vi "Teleop.vi"(10 "Match Info":T3={"Autonomous Elapsed Seconds"=0.0, "TeleOp Elapsed Seconds"=0.0, "Disabled Elapsed Seconds"=0.0, "Visited Autonomous"=FALSE, "Visited TeleOp"=FALSE, "Visited Disabled"=FALSE, "Autonomous Settings"={"Autonomous Style"=enum."Independent", "VI Refnum"=refnum}}, 11 "Call Context":T4) -> ()   [LabVIEW 2020]
doc: "This VI is called for each TeleOp packet received from the DS where the robot is not disabled. It is often used to read from the joysticks and update I/O or to update setpoints for timed control loops. It should complete and return within 20 milliseconds or it may miss DS packets."
uses:
  <vilib>/Rock Robotics/WPI/DriverStation/WPI_DriverStationDerivedRobotMode.ctl
  <vilib>/Rock Robotics/WPI/DriverStation/WPI_DriverStationMatch Info.ctl
  <vilib>/Rock Robotics/WPI/Solenoid/WPI_SolenoidValue.ctl
  <vilib>/Rock Robotics/WPI/ThirdParty/Phoenix-LabVIEW/Motor Controller/Controls/CTRE_Phoenix_MotorControl_ControlMode.ctl
  <vilib>/Rock Robotics/WPI/Utilities/WPI_GetSetVariantRefNum.vi
  <vilib>/Rock Robotics/WPI/ThirdParty/Phoenix-LabVIEW/Pigeon IMU/CTRE_PigeonIMU_GetYPR.vi
  <vilib>/Rock Robotics/Network Tables/NT Read Boolean.vi
  <vilib>/Rock Robotics/Network Tables/NT Read Number.vi
  <vilib>/Rock Robotics/Network Tables/NT Read String.vi
  <vilib>/Rock Robotics/Network Tables/NT Write Boolean.vi
  <vilib>/Rock Robotics/WPI/ThirdParty/Phoenix-LabVIEW/CANCoder/Get/CTRE_Phoenix_CANcoder_GetSensorData.vi
  <vilib>/Rock Robotics/Network Tables/NT Write String.vi
  <vilib>/Rock Robotics/WPI/Solenoid/WPI_SolenoidSetEnum.vi
  <vilib>/Rock Robotics/WPI/ThirdParty/Phoenix-LabVIEW/Motor Controller/Get/CTRE_Phoenix_MotorController_IntegratedSensorData_TalonFX.vi
  <vilib>/addons/control/pid/pid.llb/PID (DBL).vi
  <vilib>/addons/control/pid/NI_PID_pid.lvlib
panel:
  out "reject pressed":bool
  out "intake count":i32
  in  "Subtract rpm":dbl=2700.0
  out "% voltage":dbl
  out "voltage (V)":dbl
  out "Motor Volts":dbl
  out "rpm":dbl
  in  "intake start":T1=enum."Forward"
  out "limelight tx":dbl
  out "limelight ty":dbl
  in  "Elevate no want":dbl
  in  "Reject no want":dbl=-1.0
  in  "Intake no want":dbl=0.75 format="%#_13g"
  in  "Elevate wanted":dbl=-0.35
  in  "Reject wanted":dbl=1.0
  in  "Intake wanted":dbl=0.75
  out "Pigeon Value":dbl
  out "frontrightmotor":dbl
  out "frontleftdrive":dbl
  in  "PID gains 4":T2={"proportional gain (Kc)"=-0.005, "integral time (Ti, min)"=0.0, "derivative time (Td, min)"=2e-05} {"derivative time (Td, min)" format="%.6f"; "integral time (Ti, min)" format="%.6f"; "proportional gain (Kc)" format="%.6f"}
  in  "PID gains 3":T2={"proportional gain (Kc)"=0.005, "integral time (Ti, min)"=0.0, "derivative time (Td, min)"=2e-05} {"derivative time (Td, min)" format="%.6f"; "integral time (Ti, min)" format="%.6f"; "proportional gain (Kc)" format="%.6f"}
  in  "PID gains 2":T2={"proportional gain (Kc)"=-0.005, "integral time (Ti, min)"=0.0, "derivative time (Td, min)"=2e-05} {"derivative time (Td, min)" format="%.6f"; "integral time (Ti, min)" format="%.6f"; "proportional gain (Kc)" format="%.6f"}
  in  "PID gains":T2={"proportional gain (Kc)"=0.005, "integral time (Ti, min)"=0.0, "derivative time (Td, min)"=2e-05} {"derivative time (Td, min)" format="%.6f"; "integral time (Ti, min)" format="%.6f"; "proportional gain (Kc)" format="%.6f"}
  out "Motor out 4":dbl
  out "Desired Position 4":dbl
  out "Motor out 1":dbl
  out "Desired Position 1":dbl
  out "Motor Out 2":dbl
  out "Desired Position 2":dbl
  out "Motor out 3":dbl
  out "Desired Position 3":dbl
  out "Sensor Position 4":dbl
  out "Sensor Position 3":dbl
  out "Sensor Position 2":dbl
  out "Sensor Position 1":dbl
  out "Rotation steering angle 4":dbl
  out "WheelDirection4":dbl(knob) scale=180.0..-180.0
  out "Throttle 4":dbl(slide) scale=-1.0..1.0
  out "Y4":dbl
  out "X4":dbl
  out "Rotation steering angle 3":dbl
  out "WheelDirection3":dbl(knob) scale=180.0..-180.0
  out "Throttle 3":dbl(slide) scale=-1.0..1.0
  out "Y3":dbl
  out "X3":dbl
  out "Rotation steering angle 2":dbl
  out "WheelDirection2":dbl(knob) scale=180.0..-180.0
  out "Throttle 2":dbl(slide) scale=-1.0..1.0
  out "Y2":dbl
  out "X2":dbl
  out "Rotation steering angle 1":dbl
  out "WheelDirection1":dbl(knob) scale=180.0..-180.0
  out "Throttle 1":dbl(slide) scale=-1.0..1.0
  out "Y1":dbl
  out "X1":dbl
  out "Z - Axis":dbl
  out "Y - Axis":dbl
  out "X - Axis":dbl
  in  "Auto-Accept":bool
  in  "8togglePressed?":bool
  in  "Red/Blue":u32(colorbox)
  out "B":u8
  out "G":u8
  out "R":u8
  out "Color":u32(colorbox)
  out "Sample Slider 0":dbl(slide) scale=0.0..5.0
  out "Sample Boolean 1":bool
  out "Sample Boolean 0":bool
  # "-1"
  # "0"
  # ".75"
  # ".75"
  # "-.6"
  # "-.35"
  # ".1"
  # "1"
  # "-.1"
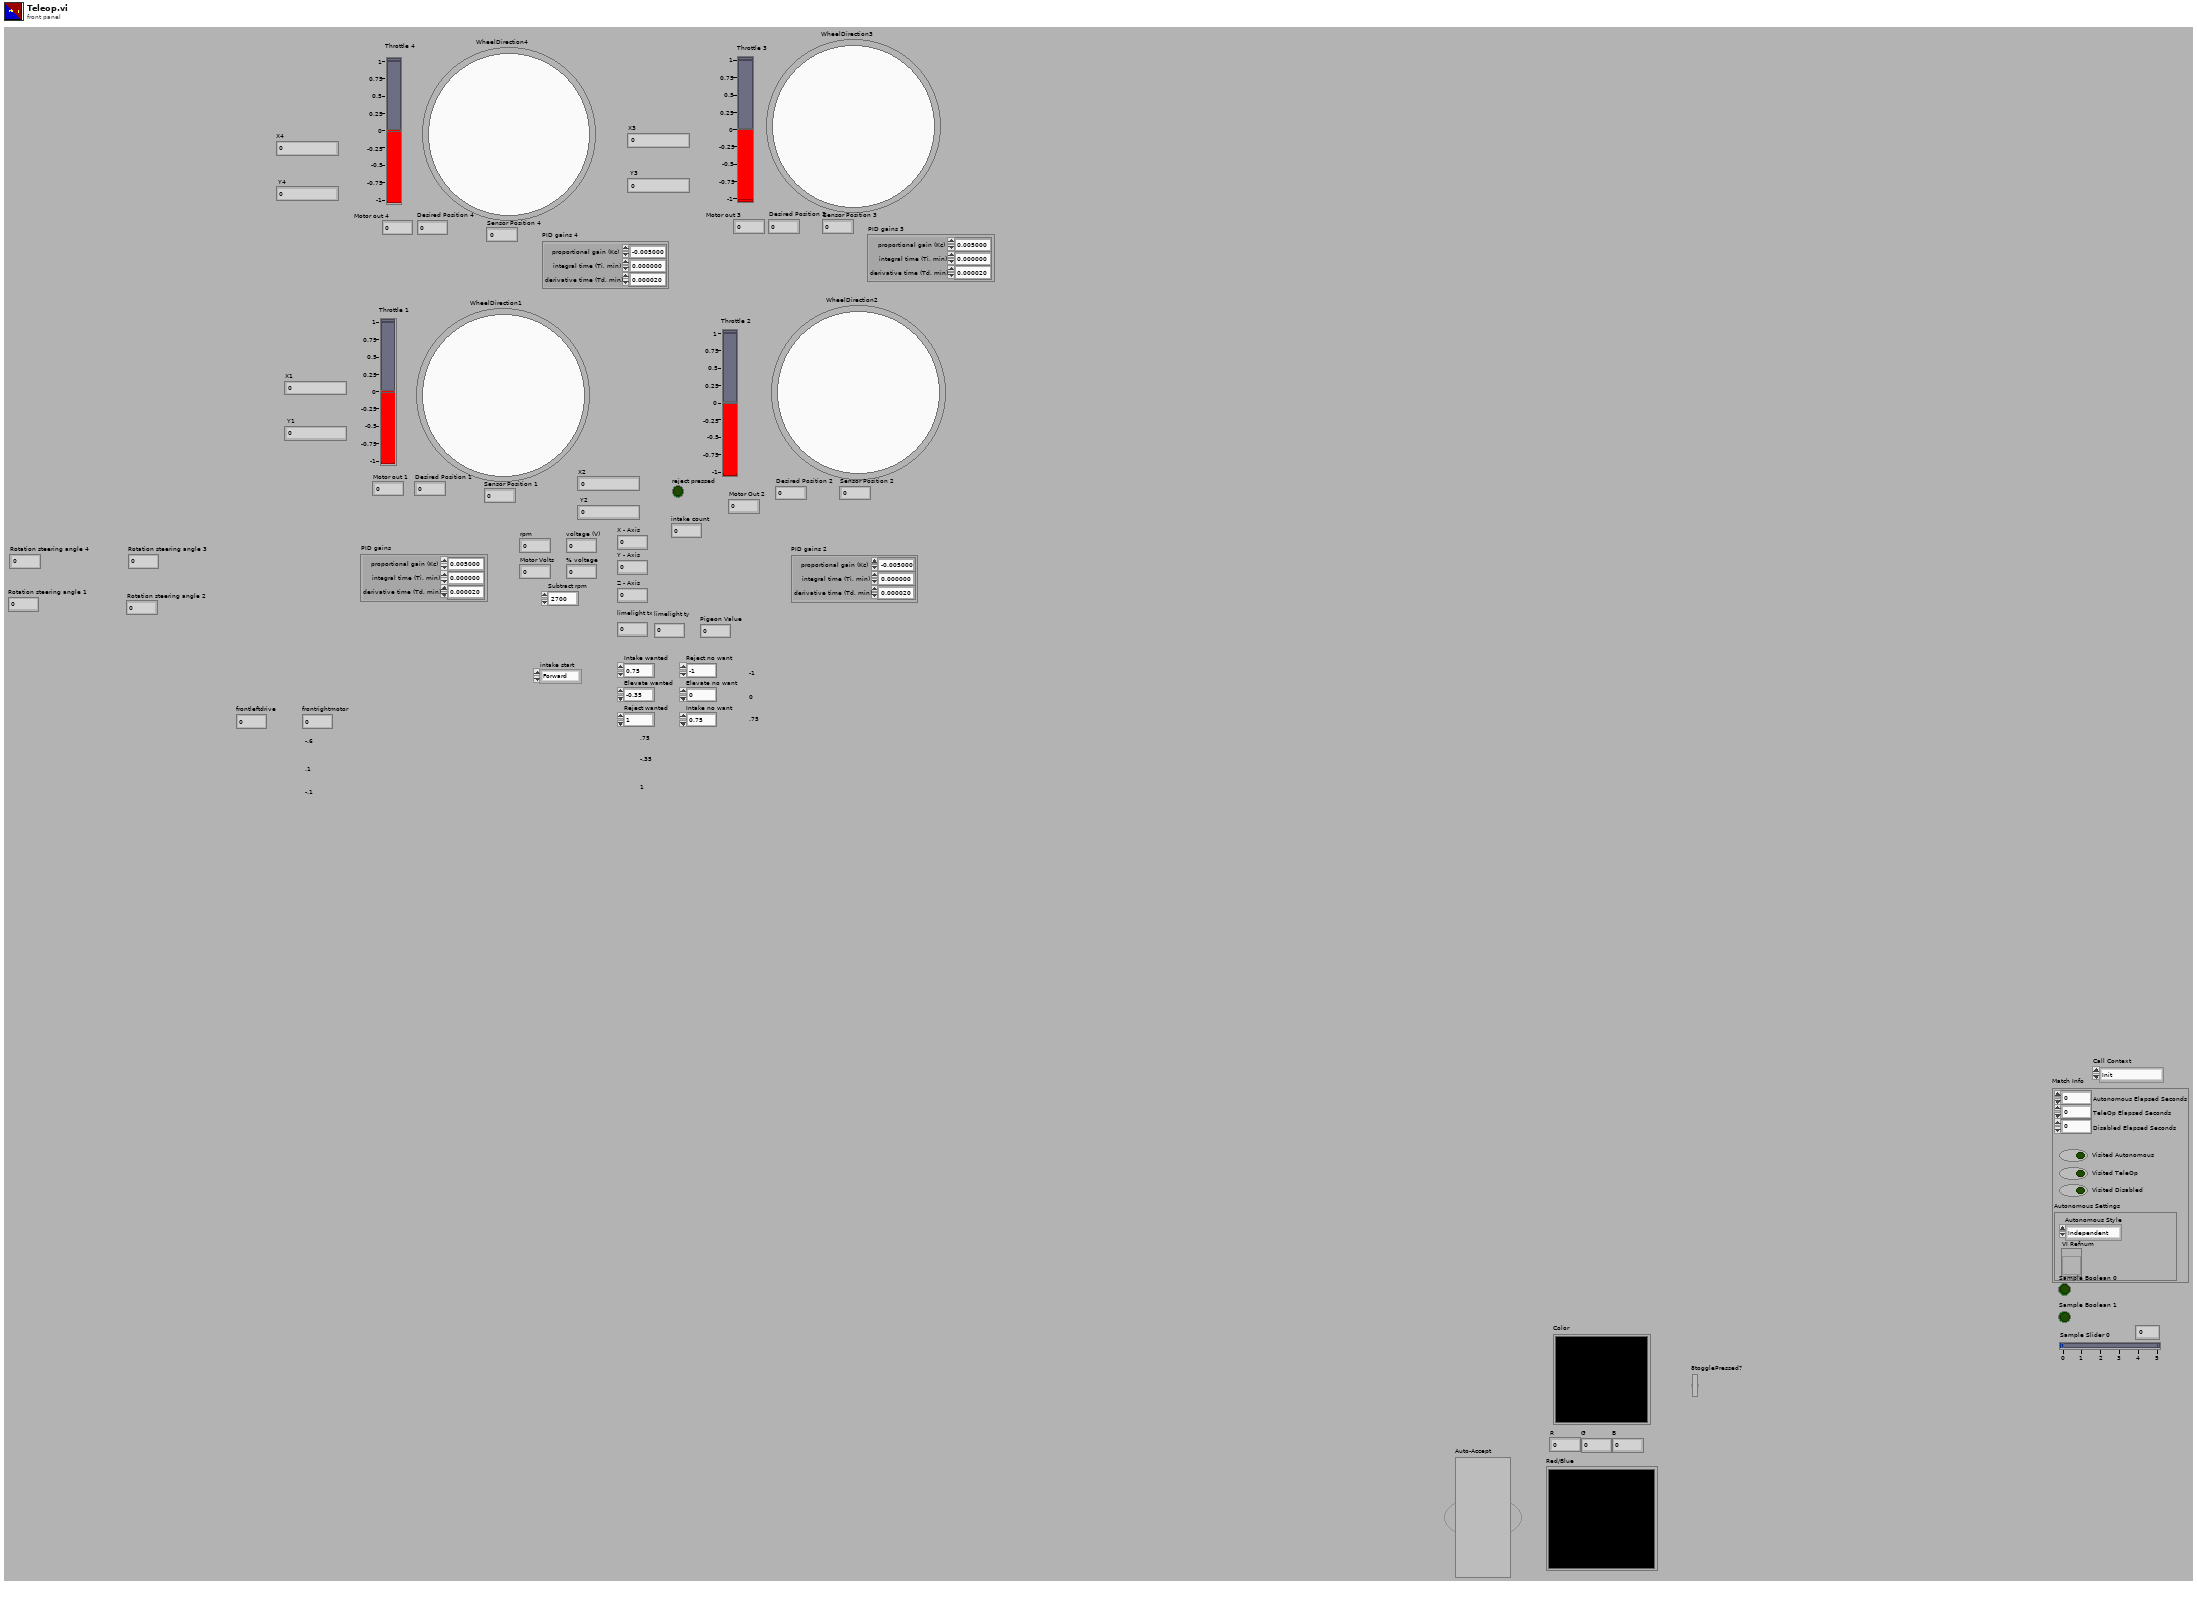
[diagram p1: front panel]
types:
  T1 = typedef "WPI_SolenoidValue.ctl" = enum16{"Off", "On", "Forward", "Reverse"}
  T2 = cluster{"proportional gain (Kc)":dbl, "integral time (Ti, min)":dbl, "derivative time (Td, min)":dbl}
  T3 = typedef "WPI_DriverStationMatch Info.ctl" = cluster{"Autonomous Elapsed Seconds":dbl, "TeleOp Elapsed Seconds":dbl, "Disabled Elapsed Seconds":dbl, "Visited Autonomous":bool, "Visited TeleOp":bool, "Visited Disabled":bool, "Autonomous Settings":cluster{"Autonomous Style":enum16{"Iterative", "Independent"}, "VI Refnum":refnum<vi>}}
  T4 = typedef "WPI_DriverStationDerivedRobotMode.ctl" = enum16{"Init", "Execute", "Stop"}
  T5 = typedef "CTRE_Phoenix_MotorControl_ControlMode.ctl" = u16
  T6 = typedef "WPI_MotorControlDeviceRef.ctl" = cluster{"DeviceStatus":errorcluster, "Type":T7, "PWM":cluster{"PWM Channel":T8, "DeadBand":T9}, "CAN":cluster{"Device Number":u8, "SetOutput VI Ref":variant, "GetOutput VI Ref":variant, "Enable VI Ref":variant, "Disable VI Ref":variant, "Data":variant}, "Invert":bool, "DIO PWM":cluster{"PWM \"Enable\" Channel":T8, "DIOChannel":T10, "PWM Rate":dbl}}
  T7 = typedef "WPI_MotorControlType.ctl" = enum16{"PWM", "CAN", "DIO PWM"}
  T8 = typedef "FPGA_DIOPWMChannel.ctl" = enum8{"PWM 0", "PWM 1", "PWM 2", "PWM 3", "PWM 4", "PWM 5", "PWM 6", "PWM 7", "PWM 8", "PWM 9", "PWM MXP 0", "PWM MXP 1", "PWM MXP 2", "PWM MXP 3", "PWM MXP 4", "PWM MXP 5", "PWM MXP 6", "PWM MXP 7", "PWM MXP 8", "PWM MXP 9", "Invalid"}
  T9 = typedef "WPI_PWMDeadband.ctl" = cluster{"Name":string, "maxPositivePwm":i32, "minPositivePwm":i32, "centerPwm":i32, "maxNegativePwm":i32, "minNegativePwm":i32, "angularRange":u16}
  T10 = typedef "FPGA_DIOChannel.ctl" = enum8{"DIO 0", "DIO 1", "DIO 2", "DIO 3", "DIO 4", "DIO 5", "DIO 6", "DIO 7", "DIO 8", "DIO 9", "DIO MXP 0", "DIO MXP 1", "DIO MXP 2", "DIO MXP 3", "DIO MXP 4", "DIO MXP 5", "DIO MXP 6", "DIO MXP 7", "DIO MXP 8", "DIO MXP 9", "DIO MXP 10", "DIO MXP 11", "DIO MXP 12", "DIO MXP 13", "DIO MXP 14", "DIO MXP 15", "SPI Port CS1", "SPI Port CS2", "SPI Port CS3", "SPI Port MISO", "SPI Port MOSI", "Invalid"}
  T11 = typedef "WPI_SolenoidDevRef.ctl" = cluster{"DevStatus":errorcluster, "Pneumatics Control Module":u8, "Forward Solenoid Channel":T12, "Reverse Solenoid Channel":T12}
  T12 = typedef "WPI_SolenoidChannel.ctl" = enum8{"Solenoid 0", "Solenoid 1", "Solenoid 2", "Solenoid 3", "Solenoid 4", "Solenoid 5", "Solenoid 6", "Solenoid 7", "Solenoid 8", "Solenoid 9", "Solenoid 10", "Solenoid 11", "Solenoid 12", "Solenoid 13", "Solenoid 14", "Solenoid 15", "Invalid"}
  T13 = typedef "WPI_CompressorDevRef.ctl" = cluster{"DevStatus":errorcluster, "Pneumatics Control Module":u8}
  T14 = typedef "WPI_SwitchDevRef.ctl" = cluster{"DevStatus":errorcluster, "DIO Channel":T10, "CntIndex":T15, "Normally Closed":bool}
  T15 = typedef "FPGA_CounterCtrSystemIndex.ctl" = enum8{"Ctr 0", "Ctr 1", "Ctr 2", "Ctr 3", "Ctr 4", "Ctr 5", "Ctr 6", "Ctr 7", "Invalid"}
  T16 = typedef "Color Sensor V3 DevRef.ctl" = cluster{"I2CDevRef":T17}
  T17 = typedef "WPI_I2CDevRef.ctl" = cluster{"DevStatus":errorcluster, "Device Address":u8, "Handle":i32, "I2C Bus":T18}
  T18 = typedef "i2c_bus.ctl" = enum16{"I2C On-Board", "I2C MXP", "Invalid"}
  T19 = typedef "WPI_JoystickDevRef.ctl" = cluster{"Device":T20}
  T20 = typedef "WPI_JoystickDeviceEnum.ctl" = enum16{"USB 0", "USB 1", "USB 2", "USB 3", "USB 4", "USB 5"}
  T21 = typedef "CTRE_PigeonIMU_DeviceRef.ctl" = cluster{"DeviceStatus":errorcluster, "Device Number":u8, "Type":T22, "Device ID":u32, "Handle":u64, "UsageFrame":u32, "Library Path":path}
  T22 = typedef "CTRE_PigeonIMU_ConnectionType.ctl" = u32
  T23 = typedef "CTRE_Phoenix_CANcoder_DeviceRef.ctl" = cluster{"DeviceStatus":errorcluster, "Device Number":u8, "Handle":u64, "UsageFrame":u32, "Library Path":path}
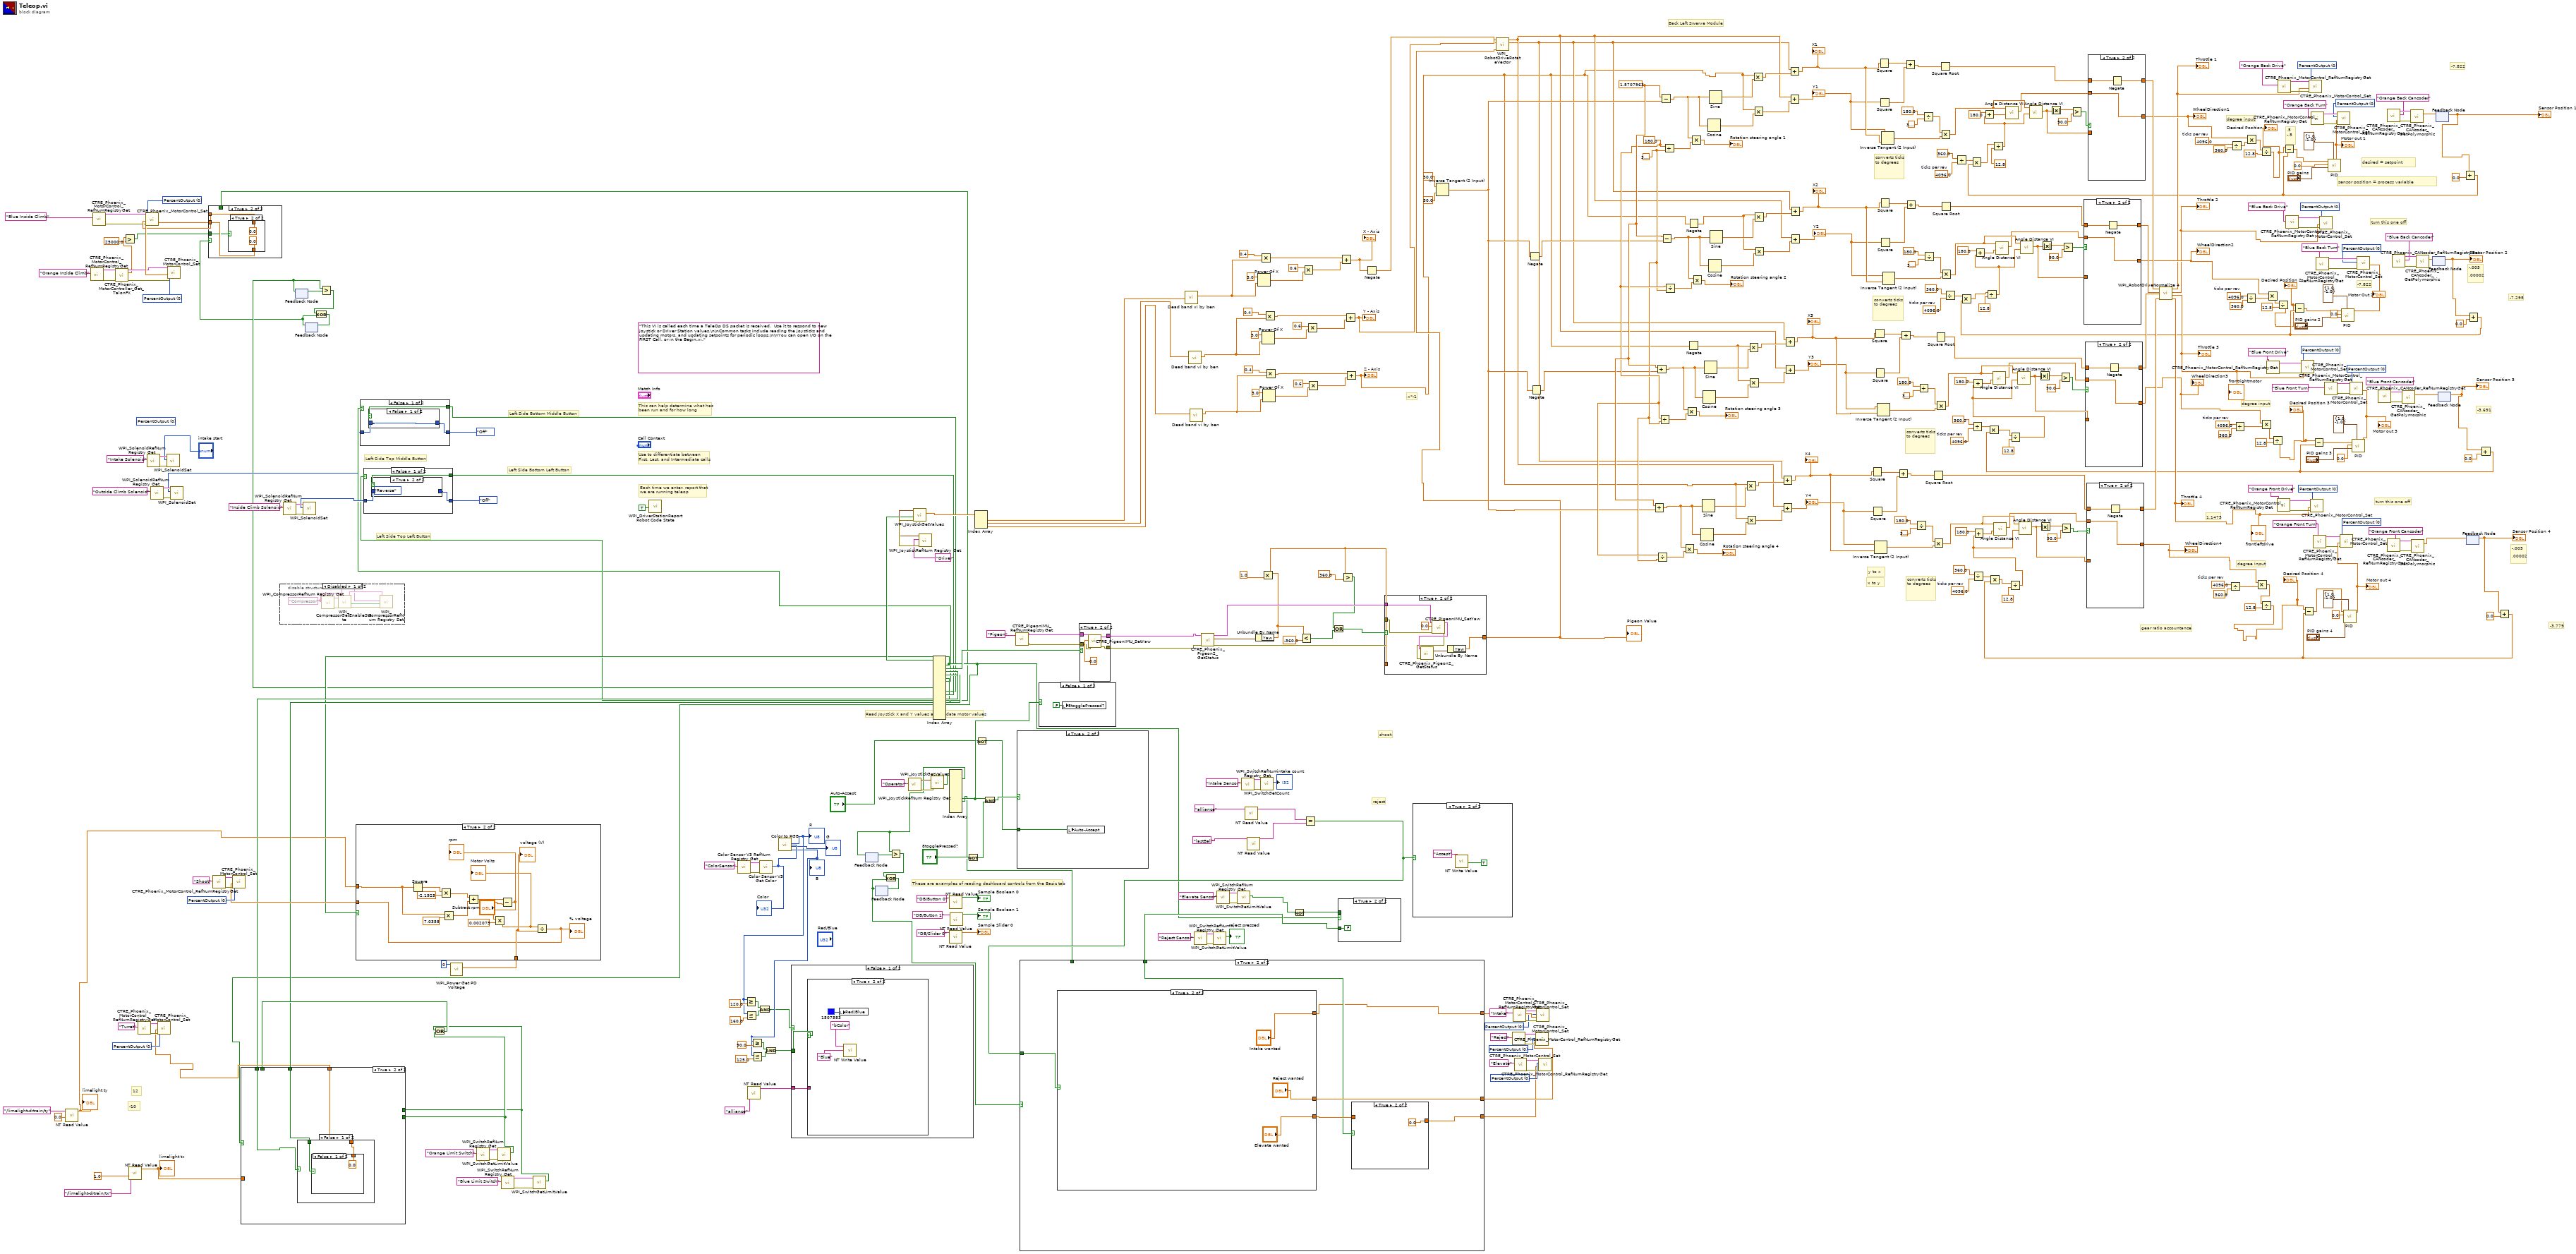
[diagram p0: block diagram]
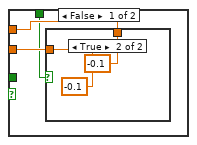
[diagram p2: hidden frame]
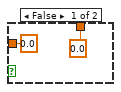
[diagram p3: hidden frame]
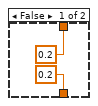
[diagram p4: hidden frame]
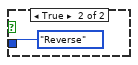
[diagram p6: hidden frame]
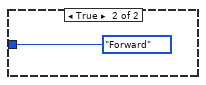
[diagram p7: hidden frame]
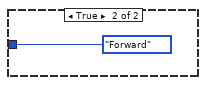
[diagram p9: hidden frame]
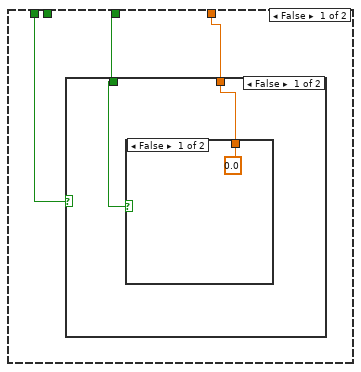
[diagram p10: hidden frame]
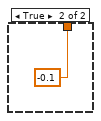
[diagram p11: hidden frame]
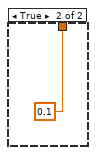
[diagram p12: hidden frame]
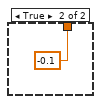
[diagram p13: hidden frame]
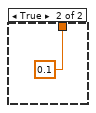
[diagram p14: hidden frame]
diagram:
  w18 = T5 0 items=["PercentOutput"=0, "Position"=1, "Velocity"=2, "Current"=3, "Follower"=5, "MotionProfile"=6, "MotionMagic"=7, "MotionProfileArc"=10, "Disabled"=15] ("Control Mode")
  w19 = T5 0 items=["PercentOutput"=0, "Position"=1, "Velocity"=2, "Current"=3, "Follower"=5, "MotionProfile"=6, "MotionMagic"=7, "MotionProfileArc"=10, "Disabled"=15] ("Control Mode")
  (unwired) T5 0 items=["PercentOutput"=0, "Position"=1, "Velocity"=2, "Current"=3, "Follower"=5, "MotionProfile"=6, "MotionMagic"=7, "MotionProfileArc"=10, "Disabled"=15] ("Control Mode")
  w88 = T5 0 items=["PercentOutput"=0, "Position"=1, "Velocity"=2, "Current"=3, "Follower"=5, "MotionProfile"=6, "MotionMagic"=7, "MotionProfileArc"=10, "Disabled"=15] ("Control Mode")
  w189 = T5 0 items=["PercentOutput"=0, "Position"=1, "Velocity"=2, "Current"=3, "Follower"=5, "MotionProfile"=6, "MotionMagic"=7, "MotionProfileArc"=10, "Disabled"=15] ("Control Mode")
  w201 = T5 0 items=["PercentOutput"=0, "Position"=1, "Velocity"=2, "Current"=3, "Follower"=5, "MotionProfile"=6, "MotionMagic"=7, "MotionProfileArc"=10, "Disabled"=15] ("Control Mode")
  w202 = T5 0 items=["PercentOutput"=0, "Position"=1, "Velocity"=2, "Current"=3, "Follower"=5, "MotionProfile"=6, "MotionMagic"=7, "MotionProfileArc"=10, "Disabled"=15] ("Control Mode")
  w203 = T5 0 items=["PercentOutput"=0, "Position"=1, "Velocity"=2, "Current"=3, "Follower"=5, "MotionProfile"=6, "MotionMagic"=7, "MotionProfileArc"=10, "Disabled"=15] ("Control Mode")
  w204 = T5 0 items=["PercentOutput"=0, "Position"=1, "Velocity"=2, "Current"=3, "Follower"=5, "MotionProfile"=6, "MotionMagic"=7, "MotionProfileArc"=10, "Disabled"=15] ("Control Mode")
  w205 = T5 0 items=["PercentOutput"=0, "Position"=1, "Velocity"=2, "Current"=3, "Follower"=5, "MotionProfile"=6, "MotionMagic"=7, "MotionProfileArc"=10, "Disabled"=15] ("Control Mode")
  w206 = T5 0 items=["PercentOutput"=0, "Position"=1, "Velocity"=2, "Current"=3, "Follower"=5, "MotionProfile"=6, "MotionMagic"=7, "MotionProfileArc"=10, "Disabled"=15] ("Control Mode")
  w207 = T5 0 items=["PercentOutput"=0, "Position"=1, "Velocity"=2, "Current"=3, "Follower"=5, "MotionProfile"=6, "MotionMagic"=7, "MotionProfileArc"=10, "Disabled"=15] ("Control Mode")
  w219 = 4096.0  # ticks per rev
  w231 = 4096.0  # ticks per rev
  w245 = 4096.0  # ticks per rev
  w256 = 4096.0  # ticks per rev
  w152 = 1.5707963 ("y")
  w265 = 4096.0  # ticks per rev
  w269 = 4096.0  # ticks per rev
  w273 = 4096.0  # ticks per rev
  w192 = 4096.0  # ticks per rev
  w150 = 3.141592653589793
  w151 = 180.0 ("x")
  w371 = T5 0 items=["PercentOutput"=0, "Position"=1, "Velocity"=2, "Current"=3, "Follower"=5, "MotionProfile"=6, "MotionMagic"=7, "MotionProfileArc"=10, "Disabled"=15] ("Control Mode")
  w387 = T5 0 items=["PercentOutput"=0, "Position"=1, "Velocity"=2, "Current"=3, "Follower"=5, "MotionProfile"=6, "MotionMagic"=7, "MotionProfileArc"=10, "Disabled"=15] ("Control Mode")
  w388 = T5 0 items=["PercentOutput"=0, "Position"=1, "Velocity"=2, "Current"=3, "Follower"=5, "MotionProfile"=6, "MotionMagic"=7, "MotionProfileArc"=10, "Disabled"=15] ("Control Mode")
  w392 = T5 0 items=["PercentOutput"=0, "Position"=1, "Velocity"=2, "Current"=3, "Follower"=5, "MotionProfile"=6, "MotionMagic"=7, "MotionProfileArc"=10, "Disabled"=15] ("Control Mode")
  (unwired) "This VI is called each time a TeleOp DS packet is received.  Use it to respond to new joystick or Driver Station values.\n\nCommon tasks include reading the joysticks and updating motors, and updating setpoints for periodic loops.\n\nYou can open I/O on the FIRST Call, or in the Begin.vi."
  # "Left Side Bottom Middle Button"
  # "Left Side Top Middle Button"
  # "Left Side Bottom Left Button"
  # "Left Side Top Left Button"
  # "shoot"
  # "reject"
  # "x*-1"
  # "12"
  # "-10"
  # ".5\n-.5"
  # "y to x"
  # "x to y"
  # "sensor position = process variable"
  # "desired = setpoint"
  # "-.005\n\n.00002"
  # "-.005\n\n.00002"
  # "-7.822"
  # "-7.295"
  # "-3.691"
  # "-3.779"
  # "1.1475"
  # "turn this one off"
  # "turn this one off"
  # "gear ratio accountance"
  # "converts ticks to degrees"
  # "converts ticks to degrees"
  # "converts ticks to degrees"
  # "converts ticks to degrees"
  # "degree input"
  # "degree input"
  # "degree input"
  # "Back Left Swerve Module"
  # "These are examples of reading dashboard controls from the Basic tab"
  # "Read Joystick X and Y values and update motor values"
  # "-7.822"
  # "Each time we enter, report that\nwe are running teleop"
  # "Use to differentiate between\nFirst, Last, and Intermediate calls"
  # "This can help determine what has\nbeen run and for how long"
  n1 = call-poly <vilib>:"NT Read Value.vi"("Default Value"=0.0, "Name"="/limelight-drtrain/ty") -> ("Numeric"=w38:dbl)  [unwired: 8 in, 1 out]
  "limelight ty" <- w38
  n2 = call <vilib>:"CTRE_Phoenix_MotorControl_RefNumRegistryGet.vi"("refnum name"="Orange Inside Climb") -> ("error out"=w15:errorcluster, "PhoenixMotorControlDevRef"=w14:T6)  [unwired: 9 in]
  n3 = call <vilib>:"CTRE_Phoenix_MotorControl_RefNumRegistryGet.vi"("refnum name"="Blue Inside Climb") -> ("error out"=w10:errorcluster, "PhoenixMotorControlDevRef"=w11:T6)  [unwired: 9 in]
  n4 = call-poly <vilib>:"CTRE_Phoenix_MotorController_Get_TalonFX.vi"("PhoenixMotorControlDevRef"=w14, "error in"=w15) -> ("PhoenixMotorControlDevRef"=w13:T6, "Position"=w3:dbl, "error out"=w12:errorcluster)  [unwired: 9 in, 2 out]
  n5 = Greater?(x=w3, y=25000.0) -> (0:w1:bool)
  n6 = call-poly <vilib>:"NT Read Value.vi"("Default Value"=1.0, "Name"="/limelight-drtrain/tx") -> ("Numeric"=w73:dbl)  [unwired: 8 in, 1 out]
  "limelight tx" <- w73
  n7 = call <vilib>:"CTRE_Phoenix_MotorControl_RefNumRegistryGet.vi"("refnum name"="Turret") -> ("error out"=w91:errorcluster, "PhoenixMotorControlDevRef"=w90:T6)  [unwired: 9 in]
  n8 = call <vilib>:"WPI_SolenoidRefNum Registry Get.vi"("refnum name"="Intake Solenoid") -> ("error out"=w77:errorcluster, "SolenoidDevRef"=w76:T11)  [unwired: 9 in]
  n9 = call <vilib>:"WPI_SolenoidRefNum Registry Get.vi"("refnum name"="Outside Climb Solenoid") -> ("error out"=w83:errorcluster, "SolenoidDevRef"=w82:T11)  [unwired: 9 in]
  n10 = call-poly <vilib>:"WPI_SolenoidSet.vi"("error in (no error)"=w77, "Value"="intake start", "SolenoidDevRef"=w76) -> ()  [unwired: 7 in, 2 out]
  n11 = call <vilib>:"CTRE_Phoenix_MotorControl_RefNumRegistryGet.vi"("refnum name"="Shoot") -> ("error out"=w374:errorcluster, "PhoenixMotorControlDevRef"=w373:T6)  [unwired: 9 in]
  n12 = disable-structure shown="Disabled" {
    frame Disabled {
      w449 = "Compressor" ("refnum name")
      n13 = call <vilib>:"WPI_CompressorRefNum Registry Get.vi"("refnum name"=w449) -> ("error out"=w454:errorcluster, "CompressorDevRef"=w453:T13)  [unwired: 9 in]
      n14 = call <vilib>:"WPI_CompressorGetEnableState.vi"("error in (no error)"=w454, "CompressorDevRef"=w453) -> ("error out"=w452:errorcluster, "Compressor Running"=w451:bool, "CompressorDevRef"=w450:T13)  [unwired: 3 in, 4 out]
      n15 = call <vilib>:"WPI_CompressorRefNum Registry Set.vi"("error in (no error)"=w452, "Test Mode Only"=w451, "refnum name"=w449, "CompressorDevRef"=w450) -> ()  [unwired: 6 in, 2 out]
    }
    frame Enabled {
    }
  }
  n16 = call <vilib>:"WPI_SolenoidRefNum Registry Get.vi"("refnum name"="Inside Climb Solenoid") -> ("error out"=w80:errorcluster, "SolenoidDevRef"=w79:T11)  [unwired: 9 in]
  n17 = feedback #1() -> (w9:bool)  [unwired: 1 in]
  n18 = feedback #2() -> (w5:bool)  [unwired: 1 in]
  n19 = call <vilib>:"WPI_Power Get PD Voltage.vi"("Power Distribution Panel (def)"=u8 0) -> ("voltage (V)"=w56:dbl)  [unwired: 13 in, 1 out]
  n20 = call <vilib>:"WPI_SwitchRefNum Registry Get.vi"("refnum name"="Orange Limit Switch") -> ("error out"=w72:errorcluster, "SwitchDevRef"=w71:T14)  [unwired: 9 in]
  n21 = call <vilib>:"WPI_SwitchGetLimitValue.vi"("error in (no error)"=w72, "SwitchDevRef"=w71) -> ("Switch Pressed"=w66:bool)  [unwired: 7 in, 2 out]
  n22 = call <vilib>:"WPI_SwitchRefNum Registry Get.vi"("refnum name"="Blue Limit Switch") -> ("error out"=w69:errorcluster, "SwitchDevRef"=w68:T14)  [unwired: 9 in]
  n23 = call <vilib>:"WPI_SwitchGetLimitValue.vi"("error in (no error)"=w69, "SwitchDevRef"=w68) -> ("Switch Pressed"=w65:bool)  [unwired: 7 in, 2 out]
  n24 = Or(x=w65, y=w66) -> (x .or. y?=w74:bool)
  n25 = call <vilib>:"WPI_DriverStationReport Robot Code State.vi"("TeleOp"=TRUE ("Autonomous")) -> ()  [unwired: 10 in, 1 out]
  n26 = call <vilib>:"Color Sensor V3 RefNum Registry Get.vi"("refnum name"="ColorSensor") -> ("error out"=w426:errorcluster, "ColorSensorDevRef"=w427:T16)  [unwired: 9 in]
  n27 = call-poly <vilib>:"NT Read Value.vi"("Name"="alliance") -> ("String"=w111:string)  [unwired: 9 in, 1 out]
  n28 = call <vilib>:"Color Sensor V3 Get Color.vi"("error in (no error)"=w426, "ColorSensorDevRef"=w427) -> ("Color"=w425:u32)  [unwired: 6 in, 3 out]
  "Color" <- w425
  n29 = call <vilib>:"Color to RGB.vi"("Color"=w425) -> ("R"=w419:u8, "G"=→"G":u8, "B"=w414:u8)  [unwired: 1 out]
  "R" <- w419
  "B" <- w414
  n30 = Greater Or Equal?(x=w419, y=120.0) -> (x >= y?=w422:bool)
  n31 = Less Or Equal?(x=w419, y=160.0) -> (x <= y?=w423:bool)
  n32 = Greater Or Equal?(x=w414, y=90.0) -> (x >= y?=w417:bool)
  n33 = Less Or Equal?(x=w414, y=125.0) -> (x <= y?=w418:bool)
  n34 = And(x=w422, y=w423) -> (x .and. y?=w403:bool)
  n35 = And(x=w417, y=w418) -> (x .and. y?=w402:bool)
  n36 = case shown="False" w403 {
    tunnel: w402 -> [w456 _]
    tunnel: w111 -> [w455 _]
    frame False {
      n37 = case shown="True" w456 {
        tunnel: w455 -> [w457 _]
        frame False {
          n38 = disable-structure shown="Disabled" {
            disable-tunnel: w457 -> [w458 _]
            frame Disabled {
              n39 = case shown="\"Blue\", Default" w458 {
                frame "Blue", Default {
                  n40 = call-poly <vilib>:"NT Write Value.vi"("String"="Red", "Name"="bColor") -> ()  [unwired: 9 in, 1 out]
                  n41 = local write "Red/Blue"(u32 16711680 ("Color Box")) -> ()
                }
                frame "Red" {
                  n42 = local write "Red/Blue"(u32 16860 ("Red/Blue")) -> ()
                  n43 = call-poly <vilib>:"NT Write Value.vi"("String"="Blue", "Name"="bColor") -> ()  [unwired: 9 in, 1 out]
                }
              }
            }
            frame Enabled {
            }
          }
        }
        frame True {
          n44 = local write "Red/Blue"(u32 1507583 ("Color Box")) -> ()
          n45 = call-poly <vilib>:"NT Write Value.vi"("String"="Blue", "Name"="bColor") -> ()  [unwired: 9 in, 1 out]
        }
      }
    }
    frame True {
      n46 = call-poly <vilib>:"NT Write Value.vi"("String"="Red", "Name"="bColor") -> ()  [unwired: 9 in, 1 out]
      n47 = local write "Red/Blue"(u32 16714752) -> ()
    }
  }
  n48 = feedback #3() -> (w379:bool)  [unwired: 1 in]
  n49 = feedback #4() -> (w375:bool)  [unwired: 1 in]
  n50 = call <vilib>:"WPI_JoystickRefNum Registry Get.vi"("refnum name"="Operator") -> ("error out"=w412:errorcluster, "JoystickDevRef"=w411:T19)  [unwired: 9 in]
  n51 = call <vilib>:"WPI_JoystickRefNum Registry Get.vi"("refnum name"="Driver") -> ("error out"=w447:errorcluster, "JoystickDevRef"=w446:T19)  [unwired: 9 in]
  n52 = call <vilib>:"WPI_JoystickGetValues.vi"("error in (no error)"=w447, "JoystickDevRef"=w446) -> ("Buttons"=w443:bool[], "Axes"=w444:dbl[])  [unwired: 5 in, 3 out]
  n53 = call <vilib>:"WPI_JoystickGetValues.vi"("error in (no error)"=w412, "JoystickDevRef"=w411) -> ("Buttons"=w410:bool[])  [unwired: 5 in, 4 out]
  n54 = Index Array(array=w443) -> (element #1=w32:bool, element #2=w440:bool, element #3=w64:bool, element #4=w63:bool, element #5=w26:bool, element #6=w24:bool, element #8=w6:bool, element #9=w23:bool, element #10=w27:bool, element #12=w4:bool)  [unwired: 17 in, 7 out]
  n55 = case shown="True" w5 {
    tunnel: [w472 w479] -> w17
    tunnel: [w473 w480] -> w16
    tunnel: w4 -> [w471 _]
    tunnel: w1 -> [_ w478]
    frame False {
      n56 = case shown="True" w471 {
        tunnel: [0.0 ("Output") -0.1 ("Output")] -> w473
        tunnel: [0.0 ("Output") -0.1 ("Output")] -> w472
        frame False {
        }
        frame True {
        }
      }
    }
    frame True {
      n57 = case shown="True" w478 {
        tunnel: [0.2 ("Output") 0.0 ("Output")] -> w480
        tunnel: [0.2 ("Output") 0.0 ("Output")] -> w479
        frame False {
        }
        frame True {
        }
      }
    }
  }
  n58 = call <vilib>:"CTRE_Phoenix_MotorControl_Set.vi"("error in (no error)"=w10, "Output"=w16, "Control Mode"=w19, "PhoenixMotorControlDevRef"=w11) -> ()  [unwired: 6 in, 2 out]
  n59 = call <vilib>:"CTRE_Phoenix_MotorControl_Set.vi"("error in (no error)"=w12, "Output"=w17, "Control Mode"=w18, "PhoenixMotorControlDevRef"=w13) -> ()  [unwired: 6 in, 2 out]
  n60 = case shown="True" w32 {
    tunnel: w74 -> [_ _]
    tunnel: w73 -> [_ _]
    tunnel: [w486 w494] -> w62
    tunnel: w66 -> [_ _]
    tunnel: w65 -> [_ _]
    tunnel: w64 -> [w487 w493]
    tunnel: w63 -> [w485 w495]
    frame False {
      n61 = case shown="False" w487 {
        tunnel: [w489 0.1 ("output")] -> w486
        tunnel: w485 -> [w488 _]
        frame False {
          n62 = case shown="False" w488 {
            tunnel: [0.0 ("output") -0.1 ("output")] -> w489
            frame False {
            }
            frame True {
            }
          }
        }
        frame True {
        }
      }
    }
    frame True {
      n63 = case shown="False" w493 {
        tunnel: [w496 0.1 ("output")] -> w494
        tunnel: w495 -> [w497 _]
        frame False {
          n64 = case shown="False" w497 {
            tunnel: [0.0 ("output") -0.1 ("output")] -> w496
            frame False {
            }
            frame True {
            }
          }
        }
        frame True {
        }
      }
    }
  }
  n65 = call <vilib>:"CTRE_Phoenix_MotorControl_Set.vi"("error in (no error)"=w91, "Output"=w62, "Control Mode"=w88, "PhoenixMotorControlDevRef"=w90) -> ()  [unwired: 6 in, 2 out]
  n66 = feedback-in #1(w6) -> ()
  n67 = Greater?(x=w6, y=w9) -> (0:w8:bool)
  n68 = Exclusive Or(1:w5, 2:w8) -> (0:w7:bool)
  n69 = feedback-in #2(w7) -> ()
  n70 = case shown="True" w32 {
    tunnel: [0.0 ("Shoot %") w503] -> w370
    tunnel: w38 -> [_ w511]
    tunnel: w56 -> [_ w505]
    frame False {
    }
    frame True {
      n71 = Square(x=w511) -> (x^2=w514:dbl)
      n72 = Multiply(x=w514, y=-2.1925) -> (x*y=w512:dbl)
      n73 = Multiply(x=w511, y=7.0358) -> (x*y=w509:dbl)
      n74 = Add(x=w512, y=w509) -> (x+y=w508:dbl)
      n75 = Subtract(x=w508, y="Subtract rpm") -> (x-y=w507:dbl)
      "rpm" <- w507
      n76 = Multiply(x=w507, y=0.002075) -> (x*y=w504:dbl)
      "Motor Volts" <- w504
      n77 = Divide(x=w504, y=w505) -> (x/y=w503:dbl)
      "% voltage" <- w503
      "voltage (V)" <- w505
    }
  }
  n78 = call <vilib>:"CTRE_Phoenix_MotorControl_Set.vi"("error in (no error)"=w374, "Output"=w370, "Control Mode"=w371, "PhoenixMotorControlDevRef"=w373) -> ()  [unwired: 6 in, 2 out]
  n79 = case shown="False" w24 {
    tunnel: [w515 WPI_SolenoidValue."Forward" ("inside climb start")] -> w22
    tunnel: WPI_SolenoidValue."Off" ("inside climb start") -> [w516 _]
    tunnel: w23 -> [w517 _]
    frame False {
      n80 = case shown="False" w517 {
        tunnel: w516 -> [w518 _]
        tunnel: [w518 WPI_SolenoidValue."Reverse" ("inside climb start")] -> w515
        frame False {
        }
        frame True {
        }
      }
    }
    frame True {
    }
  }
  n81 = call-poly <vilib>:"WPI_SolenoidSet.vi"("error in (no error)"=w83, "Value"=w22, "SolenoidDevRef"=w82) -> ()  [unwired: 7 in, 2 out]
  n82 = case shown="False" w26 {
    tunnel: [w521 WPI_SolenoidValue."Forward" ("inside climb start")] -> w29
    tunnel: WPI_SolenoidValue."Off" ("inside climb start") -> [w522 _]
    tunnel: w27 -> [w523 _]
    frame False {
      n83 = case shown="True" w523 {
        tunnel: w522 -> [w524 _]
        tunnel: [w524 WPI_SolenoidValue."Reverse" ("inside climb start")] -> w521
        frame False {
        }
        frame True {
        }
      }
    }
    frame True {
    }
  }
  n84 = call-poly <vilib>:"WPI_SolenoidSet.vi"("error in (no error)"=w80, "Value"=w29, "SolenoidDevRef"=w79) -> ()  [unwired: 7 in, 2 out]
  n85 = Index Array(array=w410) -> (element #1=w378:bool, element #7=w113:bool, element #8=w405:bool)  [unwired: 11 in, 8 out]
  n86 = feedback-in #3(w378) -> ()
  n87 = Greater?(x=w378, y=w379) -> (0:w377:bool)
  n88 = Exclusive Or(1:w375, 2:w377) -> (0:w376:bool)
  n89 = feedback-in #4(w376) -> ()
  n90 = call-poly <vilib>:"NT Read Value.vi"("Name"="DB/Button 0" ("refnum name")) -> ("Boolean"=→"Sample Boolean 0":bool)  [unwired: 9 in, 1 out]
  n91 = call-poly <vilib>:"NT Read Value.vi"("Name"="DB/Slider 0" ("refnum name")) -> ("Numeric"=→"Sample Slider 0":dbl)  [unwired: 9 in, 1 out]
  n92 = call-poly <vilib>:"NT Read Value.vi"("Name"="DB/Button 1" ("refnum name")) -> ("Boolean"=→"Sample Boolean 1":bool)  [unwired: 9 in, 1 out]
  n93 = Not(x="8togglePressed?") -> (.not. x?=w408:bool)
  n94 = Index Array(array=w444) -> (element #1=w125:dbl, element #2=w124:dbl, element #3=w123:dbl)  [unwired: 3 in]
  n95 = Not(x="Auto-Accept") -> (.not. x?=w406:bool)
  n96 = And(x=w405, y=w408) -> (x .and. y?=w407:bool)
  n97 = call <vilib>:"CTRE_PigeonIMU_RefNumRegistryGet.vi"("refnum name"="Pigeon") -> ("error out"=w441:errorcluster, "PigeonIMUDevRef"=w442:T21)  [unwired: 9 in]
  n98 = case shown="True" w407 {
    tunnel: w406 -> [_ w527]
    frame False {
    }
    frame True {
      n99 = local write "Auto-Accept"(w527) -> ()
    }
  }
  n100 = case shown="False" w405 {
    frame False {
      n101 = local write "8togglePressed?"(FALSE ("togglePressed?")) -> ()
    }
    frame True {
      n102 = local write "8togglePressed?"(TRUE ("togglePressed?")) -> ()
    }
  }
  n103 = case shown="True" w440 {
    tunnel: w442 -> [w531 w535]
    tunnel: [w531 w534] -> w436
    tunnel: w441 -> [w530 w532]
    tunnel: [w530 w533] -> w435
    frame False {
    }
    frame True {
      n104 = call <vilib>:"CTRE_PigeonIMU_SetYaw.vi"("error in (no error)"=w532, "Value"=0.0, "PigeonIMUDevRef"=w535) -> ("error out"=w533:errorcluster, "PigeonIMUDevRef"=w534:T21)  [unwired: 7 in]
    }
  }
  n105 = call "Dead band vi by ben.vi"("Numeric"=w125) -> ("Deadbanded Value"=w363:dbl)  [unwired: 10 in]
  n106 = call "Dead band vi by ben.vi"("Numeric"=w124) -> ("Deadbanded Value"=w356:dbl)  [unwired: 10 in]
  n107 = call "Dead band vi by ben.vi"("Numeric"=w123) -> ("Deadbanded Value"=w349:dbl)  [unwired: 10 in]
  n108 = call <vilib>:"WPI_SwitchRefNum Registry Get.vi"("refnum name"="Reject Sensor") -> ("error out"=w382:errorcluster, "SwitchDevRef"=w381:T14)  [unwired: 9 in]
  n109 = call-poly <vilib>:"CTRE_Phoenix_Pigeon2_GetStatus.vi"("error in (no error)"=w435, "PigeonIMUDevRef"=w436) -> ("error out"=w119:errorcluster, "Yaw Pitch Roll"=w437:cluster{"Yaw":dbl, "Pitch":dbl, "Roll":dbl}, "PigeonIMUDevRef"=w120:T21)  [unwired: 7 in]
  n110 = call <vilib>:"WPI_SwitchGetLimitValue.vi"("error in (no error)"=w382, "SwitchDevRef"=w381) -> ("Switch Pressed"=→"reject pressed":bool)  [unwired: 7 in, 2 out]
  n111 = call <vilib>:"WPI_SwitchRefNum Registry Get.vi"("refnum name"="Elevate Sensor") -> ("error out"=w37:errorcluster, "SwitchDevRef"=w36:T14)  [unwired: 9 in]
  n112 = call <vilib>:"WPI_SwitchGetLimitValue.vi"("error in (no error)"=w37, "SwitchDevRef"=w36) -> ("Switch Pressed"=w34:bool)  [unwired: 7 in, 2 out]
  n113 = call <vilib>:"WPI_SwitchRefNum Registry Get.vi"("refnum name"="Intake Sensor") -> ("error out"=w61:errorcluster, "SwitchDevRef"=w59:T14)  [unwired: 9 in]
  n114 = call-poly <vilib>:"NT Read Value.vi"("Name"="alliance") -> ("String"=w386:string)  [unwired: 9 in, 1 out]
  n115 = call-poly <vilib>:"NT Read Value.vi"("Name"="lastBall") -> ("String"=w108:string)  [unwired: 9 in, 1 out]
  n116 = Unbundle By Name(w437) -> ("Yaw"=w116:dbl)
  n117 = Power Of X(1:w363, 2:3.0 ("y")) -> (0:w367:dbl)
  n118 = Multiply(x=0.4, y=w363) -> (x*y=w364:dbl)
  n119 = call <vilib>:"WPI_SwitchGetCount.vi"("error in (no error)"=w61, "SwitchDevRef"=w59) -> ("Switch Pressed Count"=→"intake count":i32)  [unwired: 7 in, 2 out]
  n120 = Multiply(x=w116, y=1.0) -> (x*y=w121:dbl)
  n121 = Power Of X(1:w356, 2:3.0 ("y")) -> (0:w360:dbl)
  n122 = Power Of X(1:w349, 2:3.0 ("y")) -> (0:w353:dbl)
  n123 = Multiply(x=0.4, y=w356) -> (x*y=w357:dbl)
  n124 = Multiply(x=0.4, y=w349) -> (x*y=w350:dbl)
  n125 = Not(x=w34) -> (.not. x?=w33:bool)
  n126 = Less?(x=w116, y=-360.0) -> (x < y?=w117:bool)
  n127 = Multiply(x=0.6, y=w367) -> (x*y=w365:dbl)
  n128 = Equal?(x=w386, y=w108) -> (x = y?=w383:bool)
  n129 = Multiply(x=0.6, y=w360) -> (x*y=w358:dbl)
  n130 = Multiply(x=0.6, y=w353) -> (x*y=w351:dbl)
  n131 = case shown="True" w32 {
    tunnel: w33 -> [w537 _]
    tunnel: [w537 FALSE ("Switch Pressed")] -> w109
    frame False {
    }
    frame True {
    }
  }
  n132 = case shown="True" w375 {
    tunnel: [0.0 ("Intake (Reversed)") w542] -> w391
    tunnel: [0.0 ("Output") w546] -> w390
    tunnel: [0.0 ("Output") w544] -> w389
    tunnel: w383 -> [_ w547]
    tunnel: w109 -> [_ w543]
    tunnel: w113 -> [_ _]
    frame False {
    }
    frame True {
      n133 = case shown="True" w547 {
        tunnel: ["Intake no want" "Intake wanted"] -> w542
        tunnel: ["Reject no want" "Reject wanted"] -> w546
        tunnel: ["Elevate no want" "Elevate wanted"] -> w545
        frame False {
        }
        frame True {
        }
      }
      n134 = case shown="True" w543 {
        tunnel: w545 -> [w548 _]
        tunnel: [w548 0.0 ("Elevate wanted")] -> w544
        frame False {
        }
        frame True {
        }
      }
    }
  }
  n135 = Add(x=w364, y=w365) -> (x+y=w44:dbl)
  "X - Axis" <- w44
  n136 = Greater?(x=w121, y=360.0) -> (0:w118:bool)
  n137 = Or(x=w118, y=w117) -> (x .or. y?=w114:bool)
  n138 = Add(x=w357, y=w358) -> (x+y=w45:dbl)
  "Y - Axis" <- w45
  n139 = Add(x=w350, y=w351) -> (x+y=w39:dbl)
  "Z - Axis" <- w39
  n140 = Negate(x=w44) -> (-x=w42:dbl)
  n141 = case shown="True" w114 {
    tunnel: [w556 w557] -> w110
    tunnel: w121 -> [w556 _]
    tunnel: w120 -> [_ w563]
    tunnel: w119 -> [_ w562]
    frame False {
    }
    frame True {
      n142 = call <vilib>:"CTRE_PigeonIMU_SetYaw.vi"("error in (no error)"=w562, "Value"=0.0, "PigeonIMUDevRef"=w563) -> ("error out"=w558:errorcluster, "PigeonIMUDevRef"=w559:T21)  [unwired: 7 in]
      n143 = call-poly <vilib>:"CTRE_Phoenix_Pigeon2_GetStatus.vi"("error in (no error)"=w558, "PigeonIMUDevRef"=w559) -> ("Yaw Pitch Roll"=w560:cluster{"Yaw":dbl, "Pitch":dbl, "Roll":dbl})  [unwired: 7 in, 2 out]
      n144 = Unbundle By Name(w560) -> ("Yaw"=w557:dbl)
    }
  }
  "Pigeon Value" <- w110
  n145 = case shown="True" w383 {
    frame False {
      n146 = call-poly <vilib>:"NT Write Value.vi"("Boolean"=FALSE, "Name"="Accept") -> ()  [unwired: 9 in, 1 out]
    }
    frame True {
      n147 = call-poly <vilib>:"NT Write Value.vi"("Boolean"=TRUE, "Name"="Accept") -> ()  [unwired: 9 in, 1 out]
    }
  }
  n148 = Inverse Tangent (2 Input)(1:30.0 ("x"), 2:30.0 ("y")) -> (0:w142:dbl)
  n149 = call <vilib>:"WPI_RobotDriveRotateVector.vi"("Angle"=w110, "X"=w42, "Y"=w45) -> ("X'"=w43:dbl, "Y'"=w46:dbl)  [unwired: 7 out]
  n150 = call <vilib>:"CTRE_Phoenix_MotorControl_RefNumRegistryGet.vi"("refnum name"="Reject") -> ("error out"=w399:errorcluster, "PhoenixMotorControlDevRef"=w398:T6)  [unwired: 9 in]
  n151 = call <vilib>:"CTRE_Phoenix_MotorControl_RefNumRegistryGet.vi"("refnum name"="Intake") -> ("error out"=w401:errorcluster, "PhoenixMotorControlDevRef"=w400:T6)  [unwired: 9 in]
  n152 = call <vilib>:"CTRE_Phoenix_MotorControl_RefNumRegistryGet.vi"("refnum name"="Elevate") -> ("error out"=w397:errorcluster, "PhoenixMotorControlDevRef"=w396:T6)  [unwired: 9 in]
  n153 = Negate(x=w142) -> (-x=w143:dbl)
  n154 = Negate(x=w142) -> (-x=w141:dbl)
  n155 = call <vilib>:"CTRE_Phoenix_MotorControl_Set.vi"("error in (no error)"=w399, "Output"=w390, "Control Mode"=w387, "PhoenixMotorControlDevRef"=w398) -> ()  [unwired: 6 in, 2 out]
  n156 = call <vilib>:"CTRE_Phoenix_MotorControl_Set.vi"("error in (no error)"=w401, "Output"=w391, "Control Mode"=w388, "PhoenixMotorControlDevRef"=w400) -> ()  [unwired: 6 in, 2 out]
  n157 = call <vilib>:"CTRE_Phoenix_MotorControl_Set.vi"("error in (no error)"=w397, "Output"=w389, "Control Mode"=w392, "PhoenixMotorControlDevRef"=w396) -> ()  [unwired: 6 in, 2 out]
  n158 = Add(x=w152, y=w142) -> (x+y=w300:dbl)
  n159 = Add(x=w152, y=w141) -> (x+y=w313:dbl)
  n160 = Divide(x=w151, y=w150) -> (x/y=w299:dbl)
  n161 = Divide(x=w151, y=w150) -> (x/y=w312:dbl)
  n162 = Subtract(x=w152, y=w142) -> (x-y=w341:dbl)
  n163 = Subtract(x=w152, y=w143) -> (x-y=w327:dbl)
  n164 = Divide(x=w151, y=w150) -> (x/y=w340:dbl)
  n165 = Divide(x=w151, y=w150) -> (x/y=w326:dbl)
  n166 = Multiply(x=w300, y=w299) -> (x*y=→"Rotation steering angle 4":dbl)
  n167 = Multiply(x=w313, y=w312) -> (x*y=→"Rotation steering angle 3":dbl)
  n168 = Negate(x=w39) -> (-x=w40:dbl)
  n169 = Negate(x=w39) -> (-x=w41:dbl)
  n170 = Multiply(x=w341, y=w340) -> (x*y=→"Rotation steering angle 1":dbl)
  n171 = Multiply(x=w327, y=w326) -> (x*y=→"Rotation steering angle 2":dbl)
  n172 = Cosine(x=w300) -> (cos(x)=w298:dbl)
  n173 = Sine(x=w300) -> (sin(x)=w297:dbl)
  n174 = Cosine(x=w313) -> (cos(x)=w311:dbl)
  n175 = Sine(x=w313) -> (sin(x)=w310:dbl)
  n176 = Cosine(x=w341) -> (cos(x)=w338:dbl)
  n177 = Cosine(x=w327) -> (cos(x)=w324:dbl)
  n178 = Sine(x=w341) -> (sin(x)=w337:dbl)
  n179 = Sine(x=w327) -> (sin(x)=w323:dbl)
  n180 = Multiply(x=w39, y=w297) -> (x*y=w296:dbl)
  n181 = Multiply(x=w39, y=w298) -> (x*y=w295:dbl)
  n182 = Multiply(x=w40, y=w310) -> (x*y=w309:dbl)
  n183 = Multiply(x=w40, y=w311) -> (x*y=w308:dbl)
  n184 = Multiply(x=w39, y=w337) -> (x*y=w336:dbl)
  n185 = Multiply(x=w39, y=w338) -> (x*y=w335:dbl)
  n186 = Multiply(x=w41, y=w323) -> (x*y=w322:dbl)
  n187 = Multiply(x=w41, y=w324) -> (x*y=w321:dbl)
  n188 = Add(x=w43, y=w296) -> (x+y=w49:dbl)
  "X4" <- w49
  n189 = Add(x=w46, y=w295) -> (x+y=w48:dbl)
  "Y4" <- w48
  n190 = Add(x=w43, y=w309) -> (x+y=w51:dbl)
  "X3" <- w51
  n191 = Add(x=w46, y=w308) -> (x+y=w50:dbl)
  "Y3" <- w50
  n192 = Add(x=w43, y=w336) -> (x+y=w93:dbl)
  "X1" <- w93
  n193 = Add(x=w46, y=w335) -> (x+y=w92:dbl)
  "Y1" <- w92
  n194 = Add(x=w43, y=w322) -> (x+y=w95:dbl)
  "X2" <- w95
  n195 = Add(x=w46, y=w321) -> (x+y=w94:dbl)
  "Y2" <- w94
  n196 = Square(x=w49) -> (x^2=w307:dbl)
  n197 = Square(x=w48) -> (x^2=w305:dbl)
  n198 = Square(x=w51) -> (x^2=w320:dbl)
  n199 = Square(x=w50) -> (x^2=w318:dbl)
  n200 = Inverse Tangent (2 Input)(1:w49, 2:w48) -> (0:w303:dbl)
  n201 = Inverse Tangent (2 Input)(1:w51, 2:w50) -> (0:w316:dbl)
  n202 = Square(x=w93) -> (x^2=w348:dbl)
  n203 = Square(x=w92) -> (x^2=w346:dbl)
  n204 = Square(x=w95) -> (x^2=w334:dbl)
  n205 = Square(x=w94) -> (x^2=w332:dbl)
  n206 = Inverse Tangent (2 Input)(1:w93, 2:w92) -> (0:w344:dbl)
  n207 = Inverse Tangent (2 Input)(1:w95, 2:w94) -> (0:w330:dbl)
  n208 = Add(x=w307, y=w305) -> (x+y=w306:dbl)
  n209 = Add(x=w320, y=w318) -> (x+y=w319:dbl)
  n210 = Add(x=w348, y=w346) -> (x+y=w347:dbl)
  n211 = Add(x=w334, y=w332) -> (x+y=w333:dbl)
  n212 = Divide(x=180.0, y=3.141592653589793) -> (x/y=w304:dbl)
  n213 = Divide(x=180.0, y=3.141592653589793) -> (x/y=w317:dbl)
  n214 = Divide(x=180.0, y=3.141592653589793) -> (x/y=w345:dbl)
  n215 = Divide(x=180.0, y=3.141592653589793) -> (x/y=w331:dbl)
  n216 = Square Root(x=w306) -> (sqrt(x)=w214:dbl)
  n217 = Multiply(x=w304, y=w303) -> (x*y=w215:dbl)
  n218 = Square Root(x=w319) -> (sqrt(x)=w225:dbl)
  n219 = Multiply(x=w317, y=w316) -> (x*y=w227:dbl)
  n220 = Square Root(x=w347) -> (sqrt(x)=w250:dbl)
  n221 = Multiply(x=w345, y=w344) -> (x*y=w255:dbl)
  n222 = Square Root(x=w333) -> (sqrt(x)=w238:dbl)
  n223 = Multiply(x=w331, y=w330) -> (x*y=w241:dbl)
  n224 = Divide(x=360.0 ("y"), y=w245) -> (x/y=w244:dbl)
  n225 = Divide(x=360.0 ("y"), y=w256) -> (x/y=w191:dbl)
  n226 = Divide(x=360.0 ("y"), y=w231) -> (x/y=w230:dbl)
  n227 = Divide(x=360.0 ("y"), y=w219) -> (x/y=w218:dbl)
  n228 = Divide(x=w265, y=360.0) -> (x/y=w266:dbl)
  n229 = Divide(x=w192, y=360.0) -> (x/y=w277:dbl)
  n230 = Divide(x=w269, y=360.0) -> (x/y=w270:dbl)
  n231 = Divide(x=w273, y=360.0) -> (x/y=w274:dbl)
  n232 = call <vilib>:"CTRE_Phoenix_MotorControl_RefNumRegistryGet.vi"("refnum name"="Blue Front Drive") -> ("error out"=w198:errorcluster, "PhoenixMotorControlDevRef"=w290:T6)  [unwired: 9 in]
  n233 = call <vilib>:"CTRE_Phoenix_MotorControl_RefNumRegistryGet.vi"("refnum name"="Orange Front Drive") -> ("error out"=w197:errorcluster, "PhoenixMotorControlDevRef"=w287:T6)  [unwired: 9 in]
  n234 = call <vilib>:"CTRE_Phoenix_MotorControl_RefNumRegistryGet.vi"("refnum name"="Orange Back Drive") -> ("error out"=w200:errorcluster, "PhoenixMotorControlDevRef"=w294:T6)  [unwired: 9 in]
  n235 = call <vilib>:"CTRE_Phoenix_MotorControl_RefNumRegistryGet.vi"("refnum name"="Blue Back Drive") -> ("error out"=w199:errorcluster, "PhoenixMotorControlDevRef"=w291:T6)  [unwired: 9 in]
  n236 = call <vilib>:"CTRE_Phoenix_MotorControl_RefNumRegistryGet.vi"("refnum name"="Orange Back Turn") -> ("error out"=w196:errorcluster, "PhoenixMotorControlDevRef"=w285:T6)  [unwired: 9 in]
  n237 = call <vilib>:"CTRE_Phoenix_MotorControl_RefNumRegistryGet.vi"("refnum name"="Orange Front Turn") -> ("error out"=w193:errorcluster, "PhoenixMotorControlDevRef"=w282:T6)  [unwired: 9 in]
  n238 = call <vilib>:"CTRE_Phoenix_MotorControl_RefNumRegistryGet.vi"("refnum name"="Blue Back Turn") -> ("error out"=w195:errorcluster, "PhoenixMotorControlDevRef"=w284:T6)  [unwired: 9 in]
  n239 = call <vilib>:"CTRE_Phoenix_MotorControl_RefNumRegistryGet.vi"("refnum name"="Blue Front Turn") -> ("error out"=w194:errorcluster, "PhoenixMotorControlDevRef"=w283:T6)  [unwired: 9 in]
  n240 = call <vilib>:"CTRE_Phoenix_CANcoder_RefNumRegistryGet.vi"("refnum name"="Blue Front Cancoder") -> ("error out"=w181:errorcluster, "CTRE_CANcoder_DeviceRef"=w182:T23)  [unwired: 9 in]
  n241 = call <vilib>:"CTRE_Phoenix_CANcoder_RefNumRegistryGet.vi"("refnum name"="Orange Back Cancoder") -> ("error out"=w187:errorcluster, "CTRE_CANcoder_DeviceRef"=w188:T23)  [unwired: 9 in]
  n242 = call <vilib>:"CTRE_Phoenix_CANcoder_RefNumRegistryGet.vi"("refnum name"="Orange Front Cancoder") -> ("error out"=w178:errorcluster, "CTRE_CANcoder_DeviceRef"=w179:T23)  [unwired: 9 in]
  n243 = call <vilib>:"CTRE_Phoenix_CANcoder_RefNumRegistryGet.vi"("refnum name"="Blue Back Cancoder") -> ("error out"=w184:errorcluster, "CTRE_CANcoder_DeviceRef"=w185:T23)  [unwired: 9 in]
  n244 = call-poly <vilib>:"CTRE_Phoenix_CANcoder_GetPolymorphic.vi"("CTRE_CANcoder_DeviceRef"=w182, "error in"=w181) -> ("Position"=w154:dbl)  [unwired: 9 in, 4 out]
  n245 = call-poly <vilib>:"CTRE_Phoenix_CANcoder_GetPolymorphic.vi"("CTRE_CANcoder_DeviceRef"=w188, "error in"=w187) -> ("Position"=w139:dbl)  [unwired: 9 in, 4 out]
  n246 = call-poly <vilib>:"CTRE_Phoenix_CANcoder_GetPolymorphic.vi"("CTRE_CANcoder_DeviceRef"=w179, "error in"=w178) -> ("Position"=w153:dbl)  [unwired: 9 in, 4 out]
  n247 = call-poly <vilib>:"CTRE_Phoenix_CANcoder_GetPolymorphic.vi"("CTRE_CANcoder_DeviceRef"=w185, "error in"=w184) -> ("Position"=w155:dbl)  [unwired: 9 in, 4 out]
  n248 = feedback #5() -> (w138:dbl)  [unwired: 1 in]
  "Sensor Position 2" <- w138
  n249 = feedback-in #5(w155) -> ()
  n250 = feedback #6() -> (w128:dbl)  [unwired: 1 in]
  "Sensor Position 1" <- w128
  n251 = feedback-in #6(w139) -> ()
  n252 = feedback #7() -> (w136:dbl)  [unwired: 1 in]
  "Sensor Position 3" <- w136
  n253 = feedback-in #7(w154) -> ()
  n254 = Add(x=w128, y=0.0) -> (x+y=w106:dbl)
  n255 = Multiply(x=w191, y=w106) -> (x*y=w145:dbl)
  n256 = Divide(x=w145, y=12.8 ("x")) -> (x/y=w171:dbl)
  n257 = Add(x=180.0, y=w171) -> (x+y=w259:dbl)
  n258 = call "Angle Distance VI.vi"("current angle"=w259, "target angle"=w255) -> ("distance"=w251:dbl)  [unwired: 9 in]
  n259 = call "Angle Distance VI.vi"("current angle"=w171, "target angle"=w255) -> ("distance"=w252:dbl)  [unwired: 9 in]
  n260 = Absolute Value(x=w252) -> (abs(x)=w254:dbl)
  n261 = Greater?(x=w254, y=90.0 ("x")) -> (0:w176:bool)
  n262 = case shown="True" w176 {
    tunnel: w252 -> [w569 _]
    tunnel: [w569 w572] -> w190
    tunnel: w251 -> [_ w572]
    tunnel: w250 -> [w568 w571]
    tunnel: [w568 w570] -> w249
    frame False {
    }
    frame True {
      n263 = Negate(x=w571) -> (-x=w570:dbl)
    }
  }
  "WheelDirection1" <- w190
  n264 = Multiply(x=w190, y=w277) -> (x*y=w173:dbl)
  n265 = Divide(x=w173, y=12.8) -> (x/y=w55:dbl)
  "Desired Position 1" <- w55
  n266 = Subtract(x=w55, y=w106) -> (x-y=w105:dbl)
  n267 = call-poly <vilib>:"PID.vi"("output range"=cluster{"output high":dbl, "output low":dbl} {"output high"=1.0, "output low"=-1.0}, "PID gains"="PID gains", "process variable"=0.0, "setpoint"=w105) -> ("output"=w127:dbl)  [unwired: 6 in, 1 out]
  "Motor out 1" <- w127
  n268 = call <vilib>:"CTRE_Phoenix_MotorControl_Set.vi"("error in (no error)"=w196, "Output"=w127, "Control Mode"=w189, "PhoenixMotorControlDevRef"=w285) -> ()  [unwired: 6 in, 2 out]
  n269 = feedback #8() -> (w133:dbl)  [unwired: 1 in]
  "Sensor Position 4" <- w133
  n270 = feedback-in #8(w153) -> ()
  n271 = Add(x=w138, y=0.0) -> (x+y=w104:dbl)
  n272 = Multiply(x=w244, y=w104) -> (x*y=w163:dbl)
  n273 = Divide(x=w163, y=12.8) -> (x/y=w162:dbl)
  n274 = Add(x=180.0, y=w162) -> (x+y=w248:dbl)
  n275 = call "Angle Distance VI.vi"("current angle"=w248, "target angle"=w241) -> ("distance"=w239:dbl)  [unwired: 9 in]
  n276 = call "Angle Distance VI.vi"("current angle"=w162, "target angle"=w241) -> ("distance"=w236:dbl)  [unwired: 9 in]
  n277 = Absolute Value(x=w236) -> (abs(x)=w243:dbl)
  n278 = Greater?(x=w243, y=90.0 ("x")) -> (0:w240:bool)
  n279 = case shown="True" w240 {
    tunnel: w236 -> [w574 _]
    tunnel: [w574 w577] -> w235
    tunnel: w239 -> [_ w577]
    tunnel: w238 -> [w573 w576]
    tunnel: [w573 w575] -> w237
    frame False {
    }
    frame True {
      n280 = Negate(x=w576) -> (-x=w575:dbl)
    }
  }
  "WheelDirection2" <- w235
  n281 = Multiply(x=w235, y=w274) -> (x*y=w169:dbl)
  n282 = Divide(x=w169, y=12.8) -> (x/y=w54:dbl)
  "Desired Position 2" <- w54
  n283 = Subtract(x=w54, y=w104) -> (x-y=w103:dbl)
  n284 = call-poly <vilib>:"PID.vi"("output range"=cluster{"output high":dbl, "output low":dbl} {"output high"=1.0, "output low"=-1.0}, "PID gains"="PID gains 2", "process variable"=0.0, "setpoint"=w103) -> ("output"=w261:dbl)  [unwired: 6 in, 1 out]
  "Motor Out 2" <- w261
  n285 = call <vilib>:"CTRE_Phoenix_MotorControl_Set.vi"("error in (no error)"=w195, "Output"=w261, "Control Mode"=w203, "PhoenixMotorControlDevRef"=w284) -> ()  [unwired: 6 in, 2 out]
  n286 = Add(x=w136, y=0.0) -> (x+y=w101:dbl)
  n287 = Multiply(x=w230, y=w101) -> (x*y=w160:dbl)
  n288 = Divide(x=w160, y=12.8) -> (x/y=w159:dbl)
  n289 = Add(x=180.0, y=w159) -> (x+y=w234:dbl)
  n290 = call "Angle Distance VI.vi"("current angle"=w234, "target angle"=w227) -> ("distance"=w226:dbl)  [unwired: 9 in]
  n291 = call "Angle Distance VI.vi"("current angle"=w159, "target angle"=w227) -> ("distance"=w223:dbl)  [unwired: 9 in]
  n292 = Absolute Value(x=w223) -> (abs(x)=w229:dbl)
  n293 = Greater?(x=w229, y=90.0 ("x")) -> (0:w208:bool)
  n294 = case shown="True" w208 {
    tunnel: w223 -> [w579 _]
    tunnel: [w579 w582] -> w47
    tunnel: w226 -> [_ w582]
    tunnel: w225 -> [w578 w581]
    tunnel: [w578 w580] -> w224
    frame False {
    }
    frame True {
      n295 = Negate(x=w581) -> (-x=w580:dbl)
    }
  }
  "WheelDirection3" <- w47
  n296 = Multiply(x=w47, y=w270) -> (x*y=w167:dbl)
  n297 = Divide(x=w167, y=12.8) -> (x/y=w53:dbl)
  "Desired Position 3" <- w53
  n298 = Subtract(x=w53, y=w101) -> (x-y=w100:dbl)
  n299 = call-poly <vilib>:"PID.vi"("output range"=cluster{"output high":dbl, "output low":dbl} {"output high"=1.0, "output low"=-1.0}, "PID gains"="PID gains 3", "process variable"=0.0, "setpoint"=w100) -> ("output"=w262:dbl)  [unwired: 6 in, 1 out]
  "Motor out 3" <- w262
  n300 = call <vilib>:"CTRE_Phoenix_MotorControl_Set.vi"("error in (no error)"=w194, "Output"=w262, "Control Mode"=w204, "PhoenixMotorControlDevRef"=w283) -> ()  [unwired: 6 in, 2 out]
  n301 = Add(x=w133, y=0.0) -> (x+y=w97:dbl)
  n302 = Multiply(x=w218, y=w97) -> (x*y=w157:dbl)
  n303 = Divide(x=w157, y=12.8) -> (x/y=w156:dbl)
  n304 = Add(x=180.0, y=w156) -> (x+y=w222:dbl)
  n305 = call "Angle Distance VI.vi"("current angle"=w222, "target angle"=w215) -> ("distance"=w211:dbl)  [unwired: 9 in]
  n306 = call "Angle Distance VI.vi"("current angle"=w156, "target angle"=w215) -> ("distance"=w210:dbl)  [unwired: 9 in]
  n307 = Absolute Value(x=w210) -> (abs(x)=w217:dbl)
  n308 = Greater?(x=w217, y=90.0 ("x")) -> (0:w212:bool)
  n309 = case shown="True" w212 {
    tunnel: w210 -> [w584 _]
    tunnel: [w584 w587] -> w209
    tunnel: w211 -> [_ w587]
    tunnel: w214 -> [w583 w586]
    tunnel: [w583 w585] -> w213
    frame False {
    }
    frame True {
      n310 = Negate(x=w586) -> (-x=w585:dbl)
    }
  }
  "WheelDirection4" <- w209
  n311 = call <vilib>:"WPI_RobotDriveNormalize 4.vi"("D"=w213, "C"=w224, "B"=w237, "A"=w249) -> ("D'"=w129:dbl, "C'"=w286:dbl, "B'"=w130:dbl, "A'"=w126:dbl)
  "Throttle 1" <- w126
  "Throttle 2" <- w130
  "Throttle 3" <- w286
  "Throttle 4" <- w129
  "frontleftdrive" <- w129
  "frontrightmotor" <- w286
  n312 = Multiply(x=w209, y=w266) -> (x*y=w165:dbl)
  n313 = Divide(x=w165, y=12.8) -> (x/y=w52:dbl)
  "Desired Position 4" <- w52
  n314 = call <vilib>:"CTRE_Phoenix_MotorControl_Set.vi"("error in (no error)"=w198, "Output"=w286, "Control Mode"=w207, "PhoenixMotorControlDevRef"=w290) -> ()  [unwired: 6 in, 2 out]
  n315 = Subtract(x=w52, y=w97) -> (x-y=w96:dbl)
  n316 = call <vilib>:"CTRE_Phoenix_MotorControl_Set.vi"("error in (no error)"=w200, "Output"=w126, "Control Mode"=w201, "PhoenixMotorControlDevRef"=w294) -> ()  [unwired: 6 in, 2 out]
  n317 = call <vilib>:"CTRE_Phoenix_MotorControl_Set.vi"("error in (no error)"=w197, "Output"=w129, "Control Mode"=w206, "PhoenixMotorControlDevRef"=w287) -> ()  [unwired: 6 in, 2 out]
  n318 = call <vilib>:"CTRE_Phoenix_MotorControl_Set.vi"("error in (no error)"=w199, "Output"=w130, "Control Mode"=w202, "PhoenixMotorControlDevRef"=w291) -> ()  [unwired: 6 in, 2 out]
  n319 = call-poly <vilib>:"PID.vi"("output range"=cluster{"output high":dbl, "output low":dbl} {"output high"=1.0, "output low"=-1.0}, "PID gains"="PID gains 4", "process variable"=0.0, "setpoint"=w96) -> ("output"=w260:dbl)  [unwired: 6 in, 1 out]
  "Motor out 4" <- w260
  n320 = call <vilib>:"CTRE_Phoenix_MotorControl_Set.vi"("error in (no error)"=w193, "Output"=w260, "Control Mode"=w205, "PhoenixMotorControlDevRef"=w282) -> ()  [unwired: 6 in, 2 out]
